vi "WLAN - TV - RW - UTIL - CenterFrequencyToChannelNumber.vi"(0 "Center Frequency(Hz)":dbl=2407000000.0) -> (4 "Coherced Channel Number":i32, 6 "Coherced Center Frequency (Hz)":dbl)   [LabVIEW 2011]
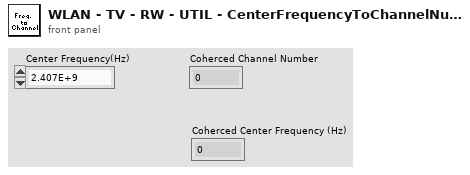
[diagram p1: front panel]
types:
  T1 = enum16{"2G Band 20M", "5G Band 20M", "5G Band 40M"}
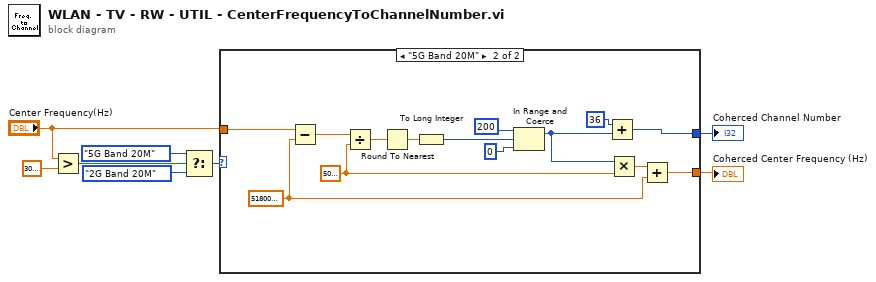
[diagram p0: block diagram]
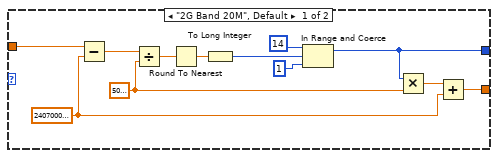
[diagram p2: hidden frame]
diagram:
  n1 = Greater?(x="Center Frequency(Hz)", y=3000000000.0) -> (0:w3:bool)
  n2 = Select(t=T1."5G Band 20M" ("Frequency Band"), s=w3, f=T1."2G Band 20M" ("Frequency Band")) -> (s? t:f=w2:T1)
  n3 = case shown="\"5G Band 20M\"" w2 {
    tunnel: "Center Frequency(Hz)" -> [w14 w29]
    tunnel: [w13 w24] -> w8
    tunnel: [w9 w25] -> w7
    frame "2G Band 20M", Default {
      w12 = 5000000.0 ("y")
      w10 = 2407000000.0 ("y")
      n4 = Subtract(x=w14, y=w10) -> (x-y=w20:dbl)
      n5 = Divide(x=w20, y=w12) -> (x/y=w19:dbl)
      n6 = Round To Nearest(number=w19) -> (nearest integer value=w17:dbl)
      n7 = To Long Integer(number=w17) -> (32bit integer=w18:i32)
      n8 = In Range and Coerce(upper limit=14, x=w18, lower limit=1) -> (coerced(x)=w13:i32)  [unwired: 1 out]
      n9 = Multiply(x=w13, y=w12) -> (x*y=w11:dbl)
      n10 = Add(x=w11, y=w10) -> (x+y=w9:dbl)
    }
    frame "5G Band 20M" {
      w28 = 5000000.0 ("y")
      w26 = 5180000000.0 ("y")
      n11 = Subtract(x=w29, y=w26) -> (x-y=w34:dbl)
      n12 = Divide(x=w34, y=w28) -> (x/y=w33:dbl)
      n13 = Round To Nearest(number=w33) -> (nearest integer value=w32:dbl)
      n14 = To Long Integer(number=w32) -> (32bit integer=w22:i32)
      n15 = In Range and Coerce(upper limit=200, x=w22, lower limit=0) -> (coerced(x)=w21:i32)  [unwired: 1 out]
      n16 = Add(x=36 ("y"), y=w21) -> (x+y=w24:i32)
      n17 = Multiply(x=w21, y=w28) -> (x*y=w27:dbl)
      n18 = Add(x=w27, y=w26) -> (x+y=w25:dbl)
    }
  }
  "Coherced Channel Number" <- w8
  "Coherced Center Frequency (Hz)" <- w7
